vi "FilterPointName.vi"(11 "RobotPoints in":string[][](array[string])) -> (0 "U":string, 1 "Z":string, 2 "Hand(V)":string, 3 "PointString out":string, 4 "Y":string, 5 "W":string, 6 "X":string)   [LabVIEW 2014]
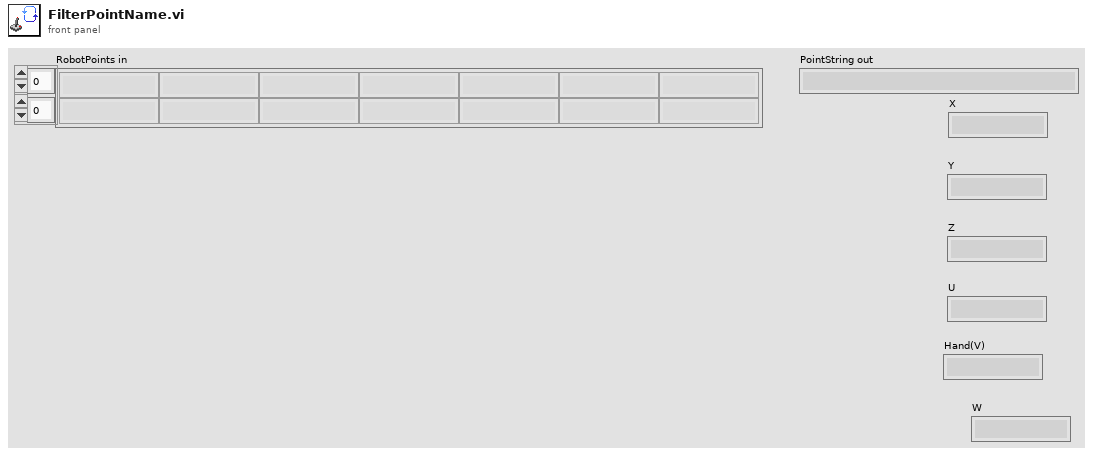
[diagram p1: front panel]
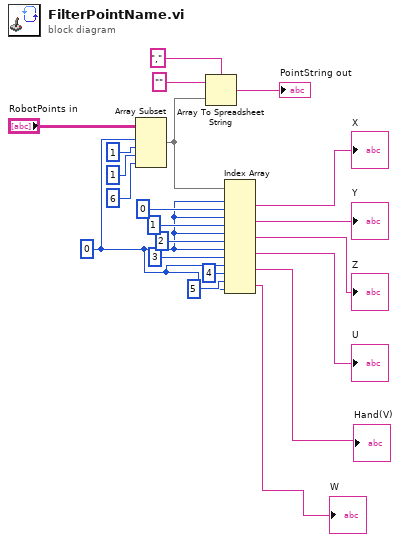
[diagram p0: block diagram]
diagram:
  w3 = 0 ("index")
  n1 = Array Subset(array="RobotPoints in", index (row)=w3, length (row)=1 ("length"), index (col)=1 ("index"), length (col)=6 ("length")) -> (w15:string[][])
  n2 = Array To Spreadsheet String(delimiter (Tab)=",", array=w15, 3:"" ("format string")) -> (spreadsheet string=→"PointString out":string)
  n3 = Index Array(array=w15, index (row) #1=w3, index (col) #1=0 ("disabled index (col)"), index (row) #2=w3, index (col) #2=1 ("disabled index (col)"), index (row) #3=w3, index (col) #3=2 ("disabled index (col)"), index (row) #4=w3, index (col) #4=3 ("disabled index (col)"), index (row) #5=w3, index (col) #5=4 ("disabled index (col)"), index (row) #6=w3, index (col) #6=5 ("disabled index (col)")) -> (element #1=→"X":string, element #2=→"Y":string, element #3=→"Z":string, element #4=→"U":string, element #5=→"Hand(V)":string, element #6=→"W":string)
